vi "create_http_communication.vi"(0 "api_key":string, 11 "error in":errorcluster) -> (4 "client handle":T1, 15 "error out":errorcluster)   [LabVIEW 2020, in "vector_qdrant.lvclass"]
uses:
  vector_qdrant.lvclass
  <vilib>/httpClient/ClientHandle.ctl
  <vilib>/httpClient/LabVIEWHTTPClient.lvlib
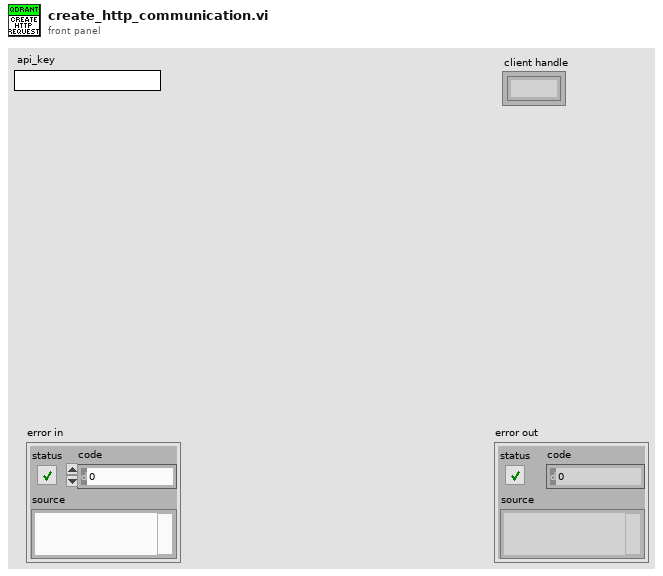
[diagram p1: front panel]
types:
  T1 = typedef "LabVIEWHTTPClient.lvlib/ClientHandle.ctl" = refnum<k1>
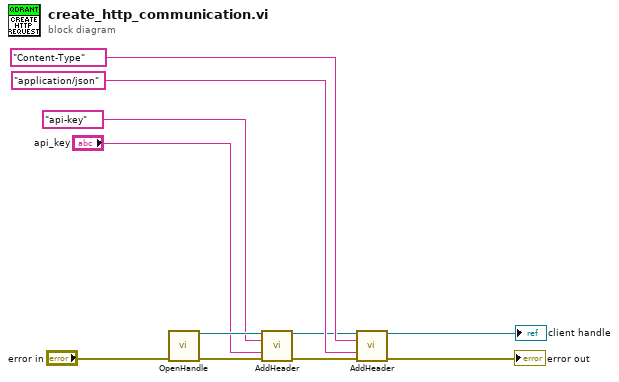
[diagram p0: block diagram]
diagram:
  n1 = call <vilib>:"OpenHandle.vi"("error in (no error)"="error in") -> ("client handle out"=w9:T1, "error out"=w10:errorcluster)  [unwired: 13 in]
  n2 = call <vilib>:"AddHeader.vi"("client handle"=w9, "header"="api-key", "value"="api_key", "error in (no error)"=w10) -> ("client handle out"=w2:T1, "error out"=w6:errorcluster)  [unwired: 10 in]
  n3 = call <vilib>:"AddHeader.vi"("client handle"=w2, "header"="Content-Type", "value"="application/json", "error in (no error)"=w6) -> ("client handle out"=→"client handle":T1, "error out"=→"error out":errorcluster)  [unwired: 10 in]
